vi "magnet position sweep and sensor read.vi"() -> ()   [LabVIEW 2012]
uses:
  <vilib>/DAQmx/read.llb/DAQmx Read (Analog 1D DBL NChan 1Samp).vi
  <vilib>/Analysis/1siggen.llb/Ramp Pattern by Samples.vi
  <vilib>/DAQmx/create/channels.llb/DAQmx Create Channel (AI-Voltage-Basic).vi
  VELMEX step motor/GMW Motion Control_VELMEX_V2_2.llb/Config.vi
  <vilib>/Utility/file.llb/Write To Spreadsheet File (DBL).vi
  <vilib>/DAQmx/miscellaneous.llb/DAQmx Fill In Error Info.vi
  <vilib>/Analysis/NI_AALBase.lvlib
panel:
  in  "file path (dialog if empty)":path
  out "transposed array":dbl[][](array[numeric])
  out "Z Position":sgl=6.0 format="%.2f"
  out "Y Position":sgl format="%.2f"
  out "X Position":sgl format="%.2f"
  out "Angle(T) Position":sgl=1.0 format="%.1f"
  in  "axis":string="T"
  in  "start":dbl format="%0.2f"
  in  "end":dbl=1.0 format="%0.2f"
  in  "samples":i32=128
  in  "GPIB Address":refnum<visa-resource-name>="GPIB0::1::INSTR"
  in  "datalog path (use dialog)":path
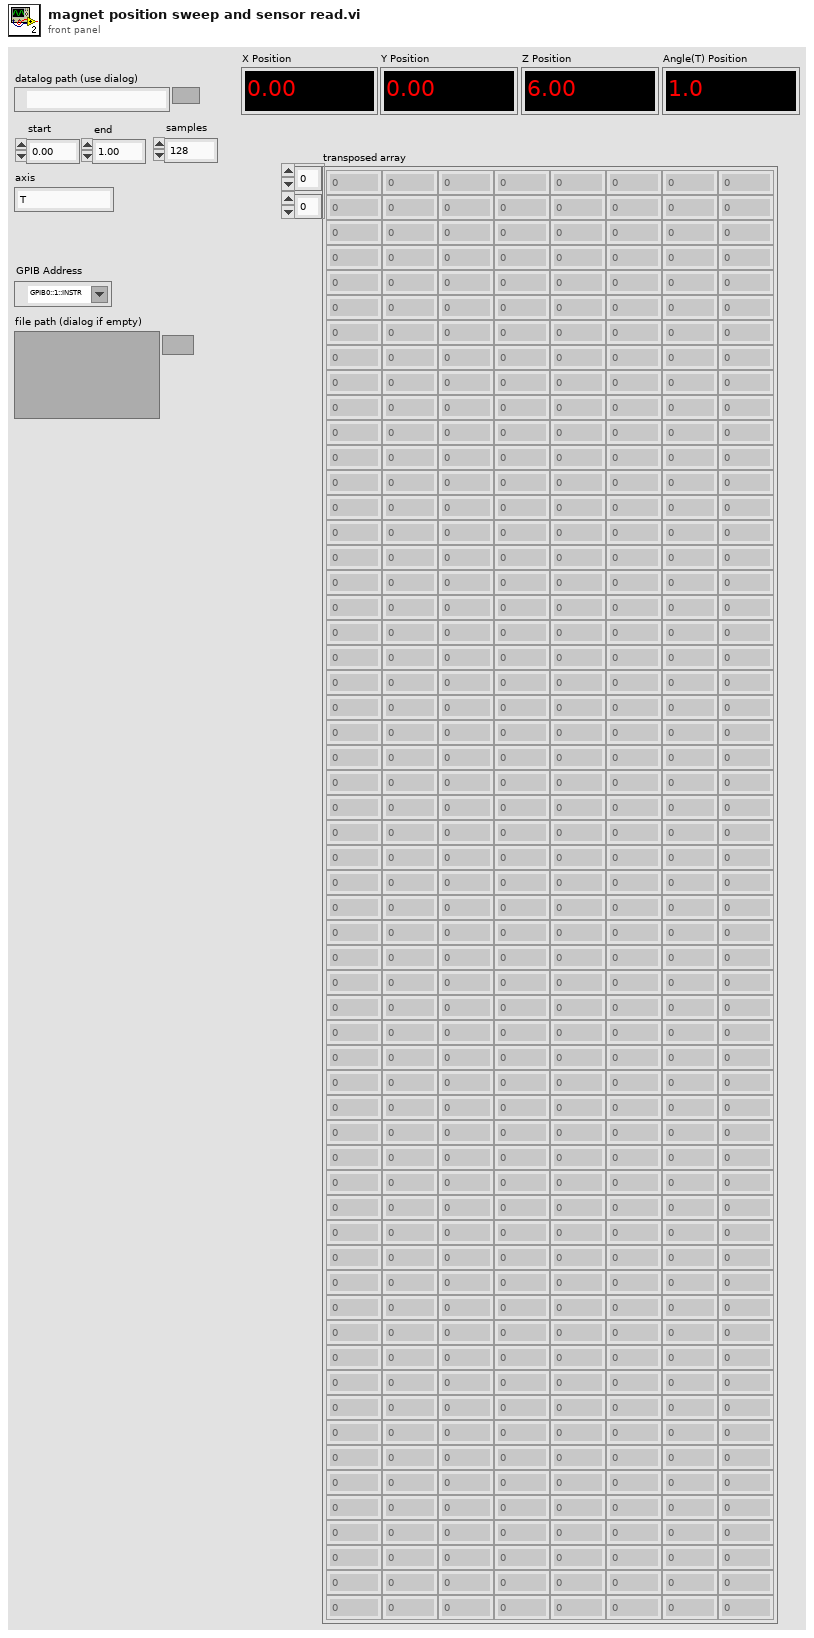
[diagram p1: front panel]
types:
  T1 = cluster{"Controller Setup":cluster{"T":string, "Z":string, "Y":string, "X":string, "CW Offset":dbl, "CCW Offset":dbl, "Z Offset":dbl, "Y Offset":dbl, "X Offset":dbl, "Rotary Resolution":i32, "Linear Resolution":i32, "T Speed":dbl, "Z Speed":dbl, "Y Speed":dbl, "X Speed":dbl}, "SoftLimit":cluster{"X soft limit":cluster{"X up soft limit":dbl, "X low soft limit":dbl}, "Y soft limit":cluster{"Y up soft limit":dbl, "Y low soft limit":dbl}, "Z soft limit":cluster{"Z up soft limit":dbl, "Z low soft limit":dbl}, "T soft limit":cluster{"T up soft limit":dbl, "T low soft limit":dbl}}}
  T2 = cluster{"T":string, "Z":string, "Y":string, "X":string, "CW Offset":dbl, "CCW Offset":dbl, "Z Offset":dbl, "Y Offset":dbl, "X Offset":dbl, "Rotary Resolution":i32, "Linear Resolution":i32, "T Speed":dbl, "Z Speed":dbl, "Y Speed":dbl, "X Speed":dbl}
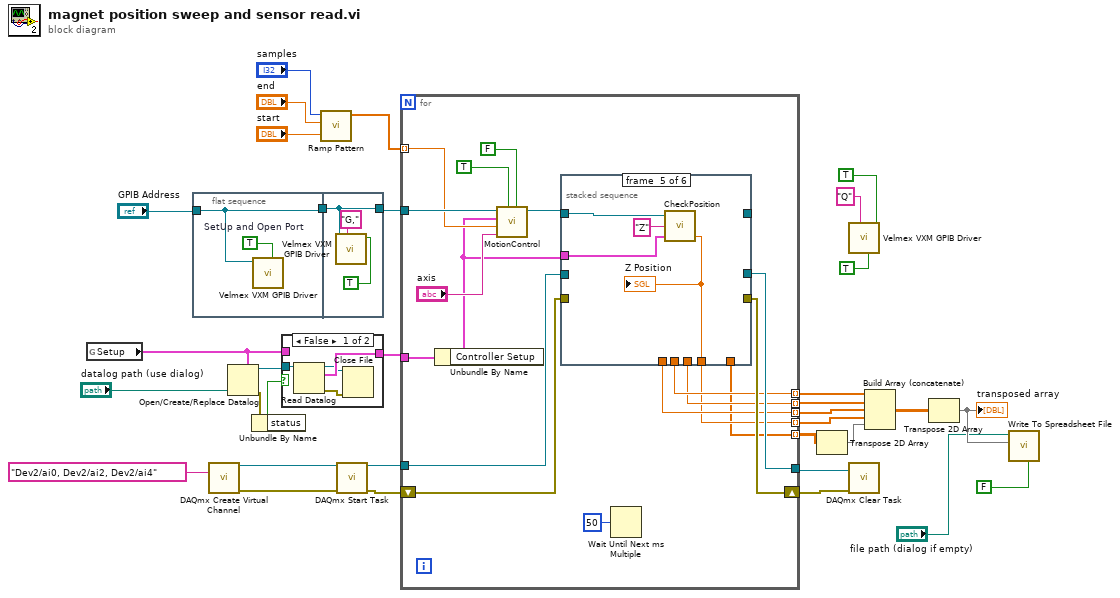
[diagram p0: block diagram]
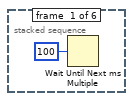
[diagram p2: hidden frame]
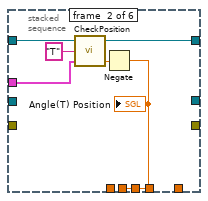
[diagram p3: hidden frame]
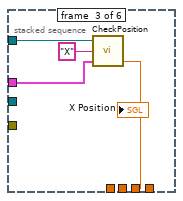
[diagram p4: hidden frame]
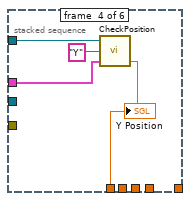
[diagram p5: hidden frame]
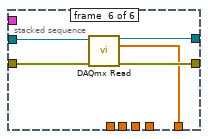
[diagram p6: hidden frame]
diagram:
  n1 = global read "Config.vi" "Setup"() -> (w31:T1)
  n2 = flat-sequence {
    tunnel: "GPIB Address" -> [w34]
    tunnel: [w34] -> w28
    tunnel: [w38] -> w23
    tunnel: w28 -> [w38]
    frame #0 {
      w35 = TRUE  # SetUp and Open Port
      n3 = call "Velmex VXM GPIB Driver.vi"("SetUp and Open Port"=w35, "VISA resource name"=w34) -> ()  [unwired: 8 in, 2 out]
    }
    frame #1 {
      n4 = call "Velmex VXM GPIB Driver.vi"("Send String to VXM"=TRUE, "String to send to VXM"="G,", "VISA resource name"=w38) -> ()  [unwired: 7 in, 2 out]
    }
  }
  n5 = call-poly <vilib>:"DAQmx Create Virtual Channel.vi"("physical channels"=tag "Dev2/ai0, Dev2/ai2, Dev2/ai4") -> ("task out"=w16:refnum<k21>, "error out"=w15:errorcluster)  [unwired: 13 in]
  n6 = Open/Create/Replace Datalog(5:w31, 11:"datalog path (use dialog)") -> (0:w33:errorcluster, 3:w32:refnum<k1>)  [unwired: 4 in, 1 out]
  n7 = Unbundle By Name(w33) -> ("status"=w30:bool)
  n8 = case shown="False" w30 {
    tunnel: w32 -> [w39 _]
    tunnel: [w42 w43] -> w22
    tunnel: w31 -> [_ w43]
    frame False {
      n9 = Read Datalog(7:w39) -> (0:w41:errorcluster, 2:w42:T1, 3:w40:refnum<k1>)  [unwired: 2 in]
      n10 = Close File(refnum=w40, error in=w41) -> ()  [unwired: 2 out]
    }
    frame True {
    }
  }
  n11 = call-poly <vilib>:"Ramp Pattern.vi"("start"="start", "end"="end", "samples"="samples") -> ("Ramp Pattern"=w18:dbl[])  [unwired: 7 in, 1 out]
  n12 = call <vilib>:"DAQmx Start Task.vi"("task/channels in"=w16, "error in"=w15) -> ("task out"=w14:refnum<k21>, "error out"=w13:errorcluster)  [unwired: 12 in]
  n13 = for {
    tunnel: w18 -> [w59] mode=indexing
    tunnel: w23 -> [w61]
    tunnel: w22 -> [w60]
    tunnel: w14 -> [w53]
    tunnel: [w51] -> w12
    shift-right: [w50] -> w11
    shift-left: w13 -> [w52]
    tunnel: [w49] -> w10 mode=indexing
    tunnel: [w48] -> w9 mode=indexing
    tunnel: [w47] -> w8 mode=indexing
    tunnel: [w46] -> w7 mode=indexing
    tunnel: [w45] -> w6 mode=indexing
    n14 = Unbundle By Name(w60) -> ("Controller Setup"=w54:T2)
    n15 = call "MotionControl.vi"("STOP motion"=FALSE, "START motion"=TRUE, "axis"="axis", "Position"=w59, "Setup"=w54, "VISA resource name in"=w61) -> ("VISA resource name out"=w55:refnum<visa-resource-name>)  [unwired: 3 in]
    n16 = stacked-sequence {
      tunnel: [_ w63 _ _ _ _] -> _
      tunnel: w55 -> [_ w67 w71 w75 w79 _]
      tunnel: w54 -> [_ w66 w70 w74 w78 _]
      tunnel: [_ w64 _ _ _ _] -> w49
      tunnel: [_ _ w69 _ _ _] -> w48
      tunnel: [_ _ _ w73 _ _] -> w47
      tunnel: [_ _ _ _ w77 _] -> w46
      tunnel: w53 -> [_ _ _ _ _ w85]
      tunnel: w52 -> [_ _ _ _ _ w84]
      tunnel: [_ _ _ _ _ w83] -> w51
      tunnel: [_ _ _ _ _ w82] -> w50
      tunnel: [_ _ _ _ _ w81] -> w45
      frame #0 {
        n17 = Wait Until Next ms Multiple(millisecond multiple=u32 100) -> ()  [unwired: 1 out]
      }
      frame #1 {
        n18 = call "CheckPosition.vi"("Setup"=w66, "Input string"="T", "VISA resource name in"=w67) -> ("Position"=w65:sgl, "VISA resource name out"=w63:refnum<visa-resource-name>)  [unwired: 1 in]
        n19 = Negate(x=w65) -> (-x=w64:sgl)
        "Angle(T) Position" <- w64
      }
      frame #2 {
        n20 = call "CheckPosition.vi"("Setup"=w70, "Input string"="X", "VISA resource name in"=w71) -> ("Position"=w69:sgl)  [unwired: 1 in, 1 out]
        "X Position" <- w69
      }
      frame #3 {
        n21 = call "CheckPosition.vi"("Setup"=w74, "Input string"="Y", "VISA resource name in"=w75) -> ("Position"=w73:sgl)  [unwired: 1 in, 1 out]
        "Y Position" <- w73
      }
      frame #4 {
        n22 = call "CheckPosition.vi"("Setup"=w78, "Input string"="Z", "VISA resource name in"=w79) -> ("Position"=w77:sgl)  [unwired: 1 in, 1 out]
        "Z Position" <- w77
      }
      frame #5 {
        n23 = call-poly <vilib>:"DAQmx Read.vi"("task/channels in"=w85, "error in"=w84) -> ("task out"=w83:refnum<k21>, "data"=w81:dbl[], "error out"=w82:errorcluster)  [unwired: 11 in]
      }
    }
    n24 = Wait Until Next ms Multiple(millisecond multiple=u32 50) -> ()  [unwired: 1 out]
  }
  n25 = Transpose 2D Array(2D array=w6) -> (transposed array=w5:dbl[][])
  n26 = call "Velmex VXM GPIB Driver.vi"("Send String to VXM"=TRUE, "Close Port"=TRUE, "String to send to VXM"="Q") -> ()  [unwired: 7 in, 2 out]
  n27 = call <vilib>:"DAQmx Clear Task.vi"("task in"=w12, "error in"=w11) -> ()  [unwired: 13 in, 1 out]
  n28 = Build Array (concatenate)(w10, w9, w8, w7, w5) -> (w4:dbl[][])
  n29 = Transpose 2D Array(2D array=w4) -> (transposed array=w3:dbl[][])
  "transposed array" <- w3
  n30 = call-poly <vilib>:"Write To Spreadsheet File.vi"("transpose? (no:F)"=FALSE, "2D data"=w3, "file path (dialog if empty)"="file path (dialog if empty)") -> ()  [unwired: 5 in, 1 out]
